vi "S2C_5190CR_Proc_Commands.vi"(7 "VI_Ref":refnum<vi>, 8 "Error In":errorcluster, 10 "Settings":T1, 11 "Q-Ref":refnum<queue>) -> (0 "Error Out":errorcluster, 2 "Stop?":bool, 3 "Response":variant)   [LabVIEW 2015]
doc: "Main VI responsible for processing all command request, both local and remote. Calls into the driver specific VIs to act on the equipment or software."
uses:
  S2C_5190CR_Proc_Globals.vi
  _Shared/S2C_Shared_Proc_Globals.vi
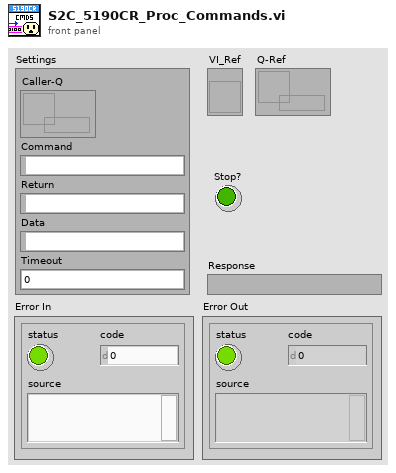
[diagram p1: front panel]
types:
  T1 = cluster{"Caller-Q":refnum<queue>, "Command":string, "Return":string, "Data":variant, "Timeout":dbl}
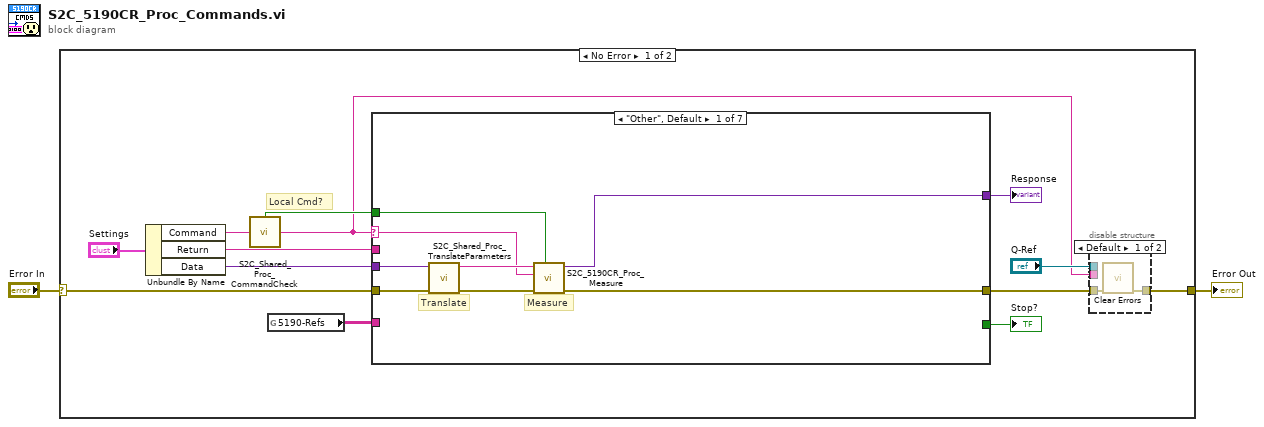
[diagram p0: block diagram]
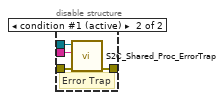
[diagram p2: hidden frame]
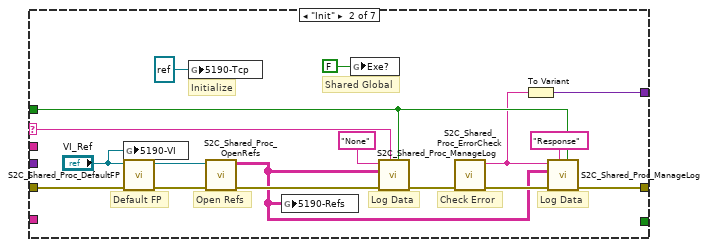
[diagram p3: hidden frame]
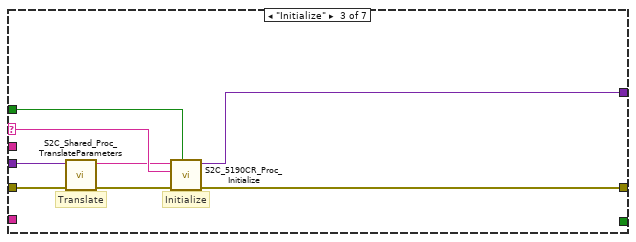
[diagram p4: hidden frame]
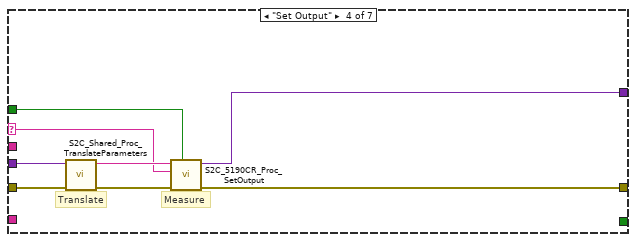
[diagram p5: hidden frame]
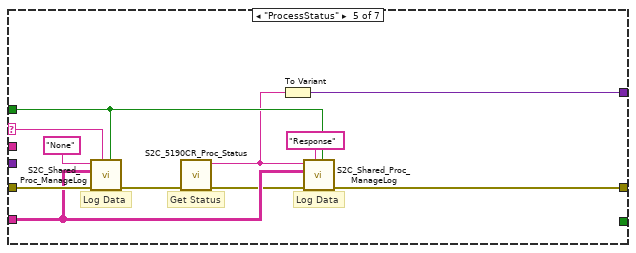
[diagram p6: hidden frame]
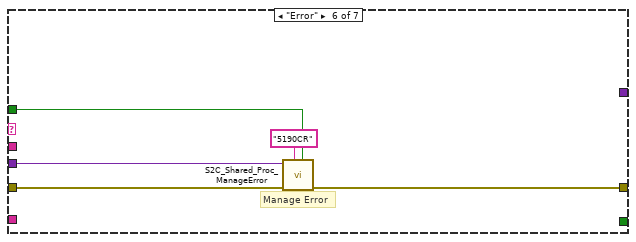
[diagram p7: hidden frame]
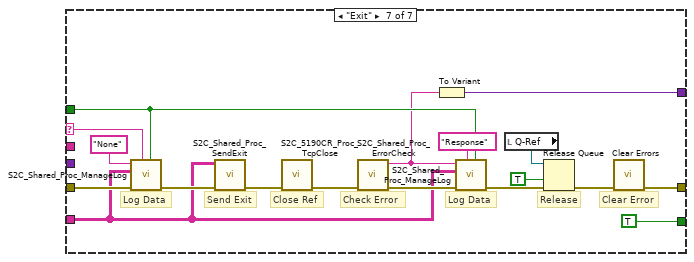
[diagram p8: hidden frame]
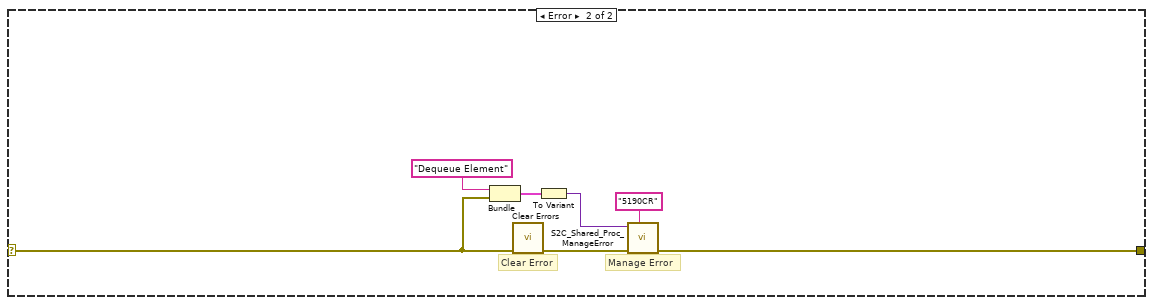
[diagram p9: hidden frame]
diagram:
  n1 = case shown="No Error" "Error In" {
    selector: "Error In" -> [w14 w98]
    tunnel: [w4 w97] -> w1
    frame No Error {
      # "Local Cmd?"
      n2 = Unbundle By Name("Settings") -> ("Command"=w8:string, "Return"=w10:string, "Data"=w15:variant)
      n3 = call "S2C_Shared_Proc_CommandCheck.vi"("Cmd In"=w8) -> ("Local?"=w7:bool, "Cmd Out"=w3:string)  [unwired: 13 in]
      n4 = global read "S2C_5190CR_Proc_Globals.vi" "5190-Refs"() -> (w9:string[][])
      n5 = case shown="\"Other\", Default" w3 {
        selector: w3 -> [w24 w43 w51 w57 w72 _ w93]
        tunnel: w14 -> [w28 w35 w54 w61 w71 w77 w94]
        tunnel: w15 -> [w27 _ w53 w60 _ w74 _]
        tunnel: [w29 w46 w52 w62 w67 w76 w80] -> w5
        tunnel: [w22 w40 w47 w55 w68 _ w88] -> w12
        tunnel: [_ _ _ _ _ _ TRUE] -> w11
        tunnel: w10 -> [_ _ _ _ _ _ _]
        tunnel: w7 -> [w23 w44 w48 w56 w70 w75 w92]
        tunnel: w9 -> [_ _ _ _ w66 _ w85]
        frame "Other", Default {
          # "Measure"
          # "Translate"
          n6 = call "S2C_Shared_Proc_TranslateParameters.vi"("Error In"=w28, "Data"=w27) -> ("Error Out"=w26:errorcluster, "JSON Cluster"=w25:string)  [unwired: 8 in]
          n7 = call "S2C_5190CR_Proc_Measure.vi"("Local?"=w23, "Error In"=w26, "Command"=w24, "JSON String"=w25) -> ("Error Out"=w29:errorcluster, "Response"=w22:variant)  [unwired: 6 in]
        }
        frame "Init" {
          # "Initialize"
          # "Default FP"
          # "Shared Global"
          # "Check Error"
          # "Log Data"
          # "Open Refs"
          # "Log Data"
          n8 = global write "S2C_5190CR_Proc_Globals.vi" "5190-VI"("VI_Ref") -> ()
          n9 = call "S2C_Shared_Proc_DefaultFP.vi"("Error In"=w35, "VI_Ref In"="VI_Ref") -> ("Error Out"=w33:errorcluster, "VI_Ref Out"=w34:refnum<vi>)  [unwired: 8 in]
          n10 = global write "S2C_5190CR_Proc_Globals.vi" "5190-Tcp"(refnum<k5> refnum ("5190-Tcp")) -> ()
          n11 = call "S2C_Shared_Proc_OpenRefs.vi"("Error In"=w33, "VI_Ref"=w34) -> ("Error Out"=w36:errorcluster, "Refs"=w32:string[][])  [unwired: 8 in]
          n12 = global write "S2C_5190CR_Proc_Globals.vi" "5190-Refs"(w32) -> ()
          n13 = global write "S2C_Shared_Proc_Globals.vi" "Exe?"(FALSE ("Exe?")) -> ()
          n14 = call "S2C_Shared_Proc_ManageLog.vi"("Local?"=w44, "Command"=w43, "Error In"=w36, "Refs"=w32, "Data In"="None") -> ("Error Out"=w38:errorcluster)  [unwired: 5 in, 1 out]
          n15 = call "S2C_Shared_Proc_ErrorCheck.vi"("Error In"=w38) -> ("Error Out"=w41:errorcluster, "Status"=w39:string)  [unwired: 9 in]
          n16 = To Variant(anything=w39) -> (Variant=w40:variant)
          n17 = call "S2C_Shared_Proc_ManageLog.vi"("Local?"=w44, "Command"="Response", "Error In"=w41, "Refs"=w32, "Data In"=w39) -> ("Error Out"=w46:errorcluster)  [unwired: 5 in, 1 out]
        }
        frame "Initialize" {
          # "Initialize"
          # "Translate"
          n18 = call "S2C_Shared_Proc_TranslateParameters.vi"("Error In"=w54, "Data"=w53) -> ("Error Out"=w50:errorcluster, "JSON Cluster"=w49:string)  [unwired: 8 in]
          n19 = call "S2C_5190CR_Proc_Initialize.vi"("Local?"=w48, "Error In"=w50, "Command"=w51, "JSON String"=w49) -> ("Error Out"=w52:errorcluster, "Response"=w47:variant)  [unwired: 6 in]
        }
        frame "Set Output" {
          # "Measure"
          # "Translate"
          n20 = call "S2C_Shared_Proc_TranslateParameters.vi"("Error In"=w61, "Data"=w60) -> ("Error Out"=w59:errorcluster, "JSON Cluster"=w58:string)  [unwired: 8 in]
          n21 = call "S2C_5190CR_Proc_SetOutput.vi"("Local?"=w56, "Error In"=w59, "Command"=w57, "JSON String"=w58) -> ("Error Out"=w62:errorcluster, "Response"=w55:variant)  [unwired: 6 in]
        }
        frame "ProcessStatus" {
          # "Get Status"
          # "Log Data"
          # "Log Data"
          n22 = call "S2C_Shared_Proc_ManageLog.vi"("Local?"=w70, "Command"=w72, "Error In"=w71, "Refs"=w66, "Data In"="None") -> ("Error Out"=w65:errorcluster)  [unwired: 5 in, 1 out]
          n23 = call "S2C_5190CR_Proc_Status.vi"("Error In"=w65) -> ("Error Out"=w64:errorcluster, "Response"=w63:string)  [unwired: 9 in]
          n24 = To Variant(anything=w63) -> (Variant=w68:variant)
          n25 = call "S2C_Shared_Proc_ManageLog.vi"("Local?"=w70, "Command"="Response", "Error In"=w64, "Refs"=w66, "Data In"=w63) -> ("Error Out"=w67:errorcluster)  [unwired: 5 in, 1 out]
        }
        frame "Error" {
          # "Manage Error"
          n26 = call "S2C_Shared_Proc_ManageError.vi"("Local?"=w75, "Process"="5190CR", "Error In"=w77, "Data"=w74) -> ("Error Out"=w76:errorcluster)  [unwired: 7 in]
        }
        frame "Exit" {
          # "Clear Error"
          # "Release"
          # "Close Ref"
          # "Check Error"
          # "Send Exit"
          # "Log Data"
          # "Log Data"
          n27 = call "S2C_Shared_Proc_ManageLog.vi"("Local?"=w92, "Command"=w93, "Error In"=w94, "Refs"=w85, "Data In"="None") -> ("Error Out"=w86:errorcluster)  [unwired: 5 in, 1 out]
          n28 = call "S2C_Shared_Proc_SendExit.vi"("Error In"=w86, "Refs"=w85) -> ("Error Out"=w84:errorcluster)  [unwired: 9 in]
          n29 = call "S2C_5190CR_Proc_TcpClose.vi"("Error In"=w84) -> ("Error Out"=w83:errorcluster)  [unwired: 10 in]
          n30 = call "S2C_Shared_Proc_ErrorCheck.vi"("Error In"=w83) -> ("Error Out"=w90:errorcluster, "Status"=w87:string)  [unwired: 9 in]
          n31 = To Variant(anything=w87) -> (Variant=w88:variant)
          n32 = call "S2C_Shared_Proc_ManageLog.vi"("Local?"=w92, "Command"="Response", "Error In"=w90, "Refs"=w85, "Data In"=w87) -> ("Error Out"=w89:errorcluster)  [unwired: 5 in, 1 out]
          n33 = local read "Q-Ref"() -> (w81:refnum<queue>)
          n34 = Release Queue(queue=w81, force destroy? (F)=TRUE, error in (no error)=w89) -> (error out=w82:errorcluster)  [unwired: 2 out]
          n35 = call <vilib>:"Clear Errors.vi"("error in (no error)"=w82) -> ("error out"=w80:errorcluster)  [unwired: 5 in, 1 out]
        }
      }
      "Response" <- w12
      "Stop?" <- w11
      n36 = disable-structure shown="Default" {
        disable-tunnel: w5 -> [w17 w21]
        disable-tunnel: [w16 w20] -> w4
        disable-tunnel: w3 -> [_ w19]
        disable-tunnel: "Q-Ref" -> [_ w18]
        frame condition #0 {
          n37 = call <vilib>:"Clear Errors.vi"("error in (no error)"=w17) -> ("error out"=w16:errorcluster)  [unwired: 5 in, 1 out]
        }
        frame condition #1 (active) {
          # "Error Trap"
          n38 = call "S2C_Shared_Proc_ErrorTrap.vi"("Error In"=w21, "Command"=w19, "Q-Ref"=w18) -> ("Error Out"=w20:errorcluster)  [unwired: 8 in]
        }
      }
    }
    frame Error {
      # "Clear Error"
      # "Manage Error"
      n39 = Bundle("Dequeue Element", "error IO"=w98) -> (w102:cluster{string, "error IO":errorcluster})  [unwired: 1 in]
      n40 = call <vilib>:"Clear Errors.vi"("error in (no error)"=w98) -> ("error out"=w99:errorcluster)  [unwired: 5 in, 1 out]
      n41 = To Variant(anything=w102) -> (Variant=w100:variant)
      n42 = call "S2C_Shared_Proc_ManageError.vi"("Process"="5190CR", "Error In"=w99, "Data"=w100) -> ("Error Out"=w97:errorcluster)  [unwired: 8 in]
    }
  }
  "Error Out" <- w1
